vi "GRAPH.vi"() -> ()   [LabVIEW 2017]
uses:
  <vilib>/Utility/miscctls.llb/LVPointDoubleTypeDef.ctl
  <vilib>/measure/NI_MAPro.lvlib
panel:
  in  "peaks/valleys":u16(ring) items=["Peaks", "Valleys"]
  in  "width":i32=3
  out "# found":i32
  out "Array 2":ext[](array[numeric])
  in  "threshold":dbl=130.0 format="%#_13g"
  out "size(s) 3":i32
  out "2nd Derivatives":dbl[](array[numeric]) format="%0.2f"
  out "Amplitudes":dbl[](array[numeric]) format="%0.2f"
  out "Locations":dbl[](array[numeric]) format="%0.2f"
  out "time stamp":timestamp[](array[timestamp])
  out "XY Graph 2":cluster{"time stamp":timestamp, "X":dbl}[](graph)
  out "number":ext[](array[numeric])
  # "GRAPH"
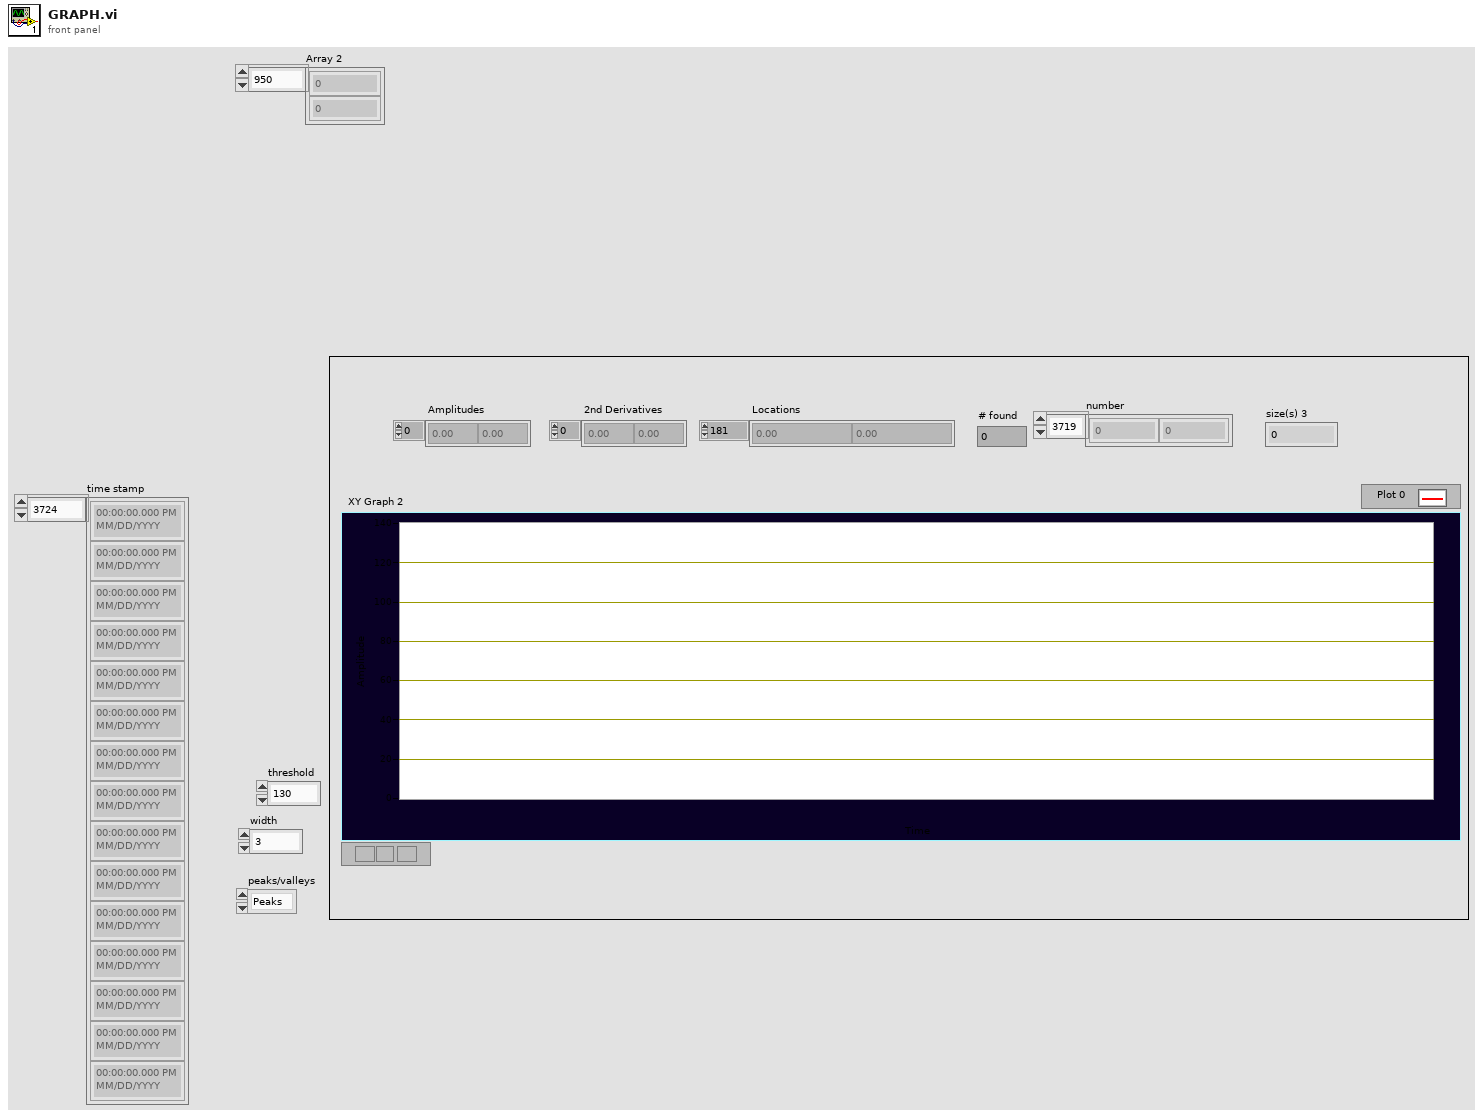
[diagram p1: front panel]
types:
  T1 = typedef "LVPointDoubleTypeDef.ctl" = cluster{"X":dbl, "Y":dbl}
  T2 = typedef "LVDateTimeRec.ctl" = cluster{"fractional second":dbl, "second":i32, "minute":i32, "hour":i32, "day of month":i32, "month":i32, "year":i32, "day of week":i32, "day of year":i32, "DST":i32}
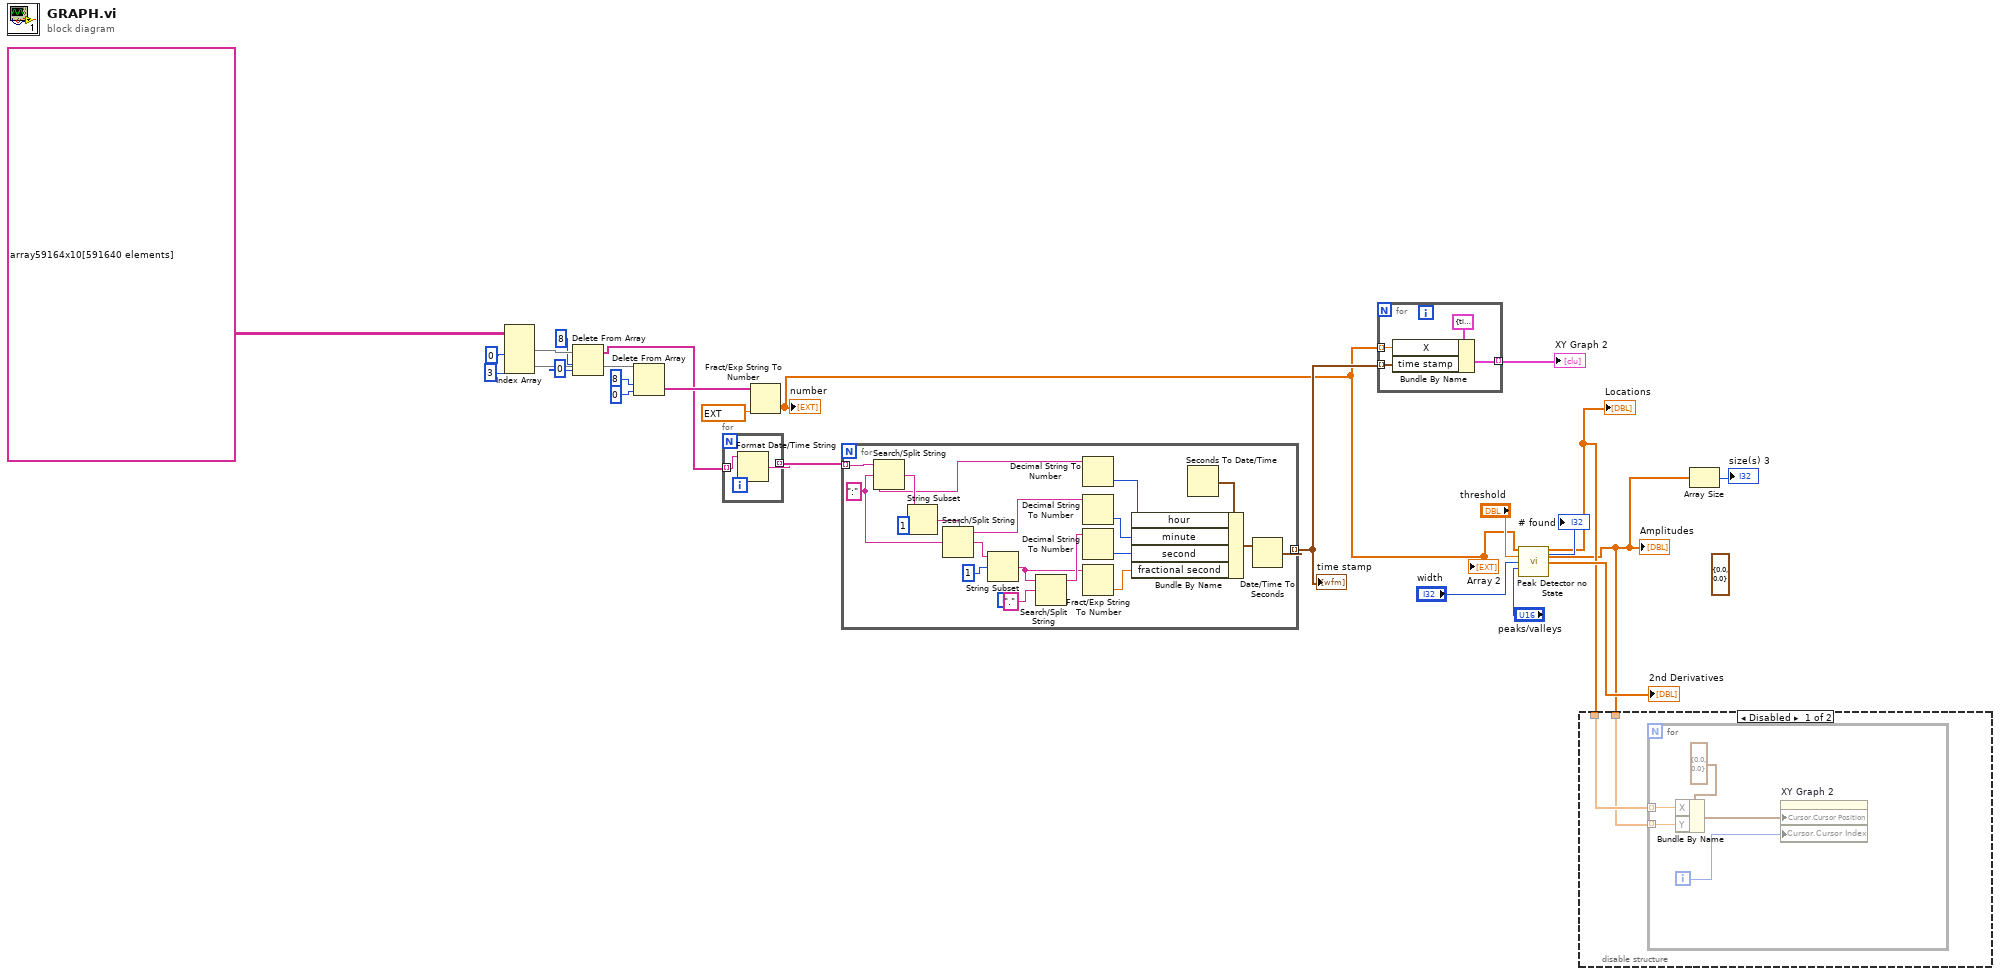
[diagram p0: block diagram]
diagram:
  (unwired) T1 {"X"=0.0, "Y"=0.0} ("Cursor.Cursor Position")
  n1 = Index Array(array=string[][] array59164x10[591640 elements] ("all rows 2"), index (col) #1=0 ("index (row)"), index (col) #2=3 ("disabled index (col)")) -> (element #1=w24:string[], element #2=w20:string[])  [unwired: 2 in]
  n2 = Delete From Array(array=w24, length=8 ("index (row)"), index=0 ("index (row)")) -> (array with subset deleted=w14:string[])  [unwired: 1 out]
  n3 = Delete From Array(array=w20, length=8 ("index (row)"), index=0 ("index (row)")) -> (array with subset deleted=w15:string[])  [unwired: 1 out]
  n4 = for {
    tunnel: w14 -> [w26] mode=indexing
    tunnel: [w25] -> w13 mode=indexing
    n5 = Format Date/Time String(time format string (%c)=w26) -> (date/time string=w25:string)  [unwired: 2 in]
  }
  n6 = Fract/Exp String To Number(string=w15, default (0 dbl)=ext 0.0 ("String")) -> (number=w5:ext[])  [unwired: 2 in, 1 out]
  "number" <- w5
  "Array 2" <- w5
  n7 = for {
    tunnel: w13 -> [w35] mode=indexing
    tunnel: [w43] -> w12 mode=indexing
    w42 = ":" ("format string")
    n8 = Search/Split String(string=w35, search string/char (-)=w42) -> (substring before match=w31:string, match + rest of string=w40:string)  [unwired: 1 in, 1 out]
    n9 = String Subset(string=w40, offset (0)=1) -> (substring=w39:string)  [unwired: 1 in]
    n10 = Search/Split String(string=w39, search string/char (-)=w42) -> (substring before match=w30:string, match + rest of string=w37:string)  [unwired: 1 in, 1 out]
    n11 = String Subset(string=w37, offset (0)=1) -> (substring=w29:string)  [unwired: 1 in]
    n12 = Search/Split String(string=w29, search string/char (-)="." ("format string")) -> (substring before match=w34:string)  [unwired: 1 in, 2 out]
    n13 = Decimal String To Number(string=w31) -> (number=w32:i32)  [unwired: 2 in, 1 out]
    n14 = Decimal String To Number(string=w30) -> (number=w33:i32)  [unwired: 2 in, 1 out]
    n15 = Decimal String To Number(string=w34) -> (number=w27:i32)  [unwired: 2 in, 1 out]
    n16 = Fract/Exp String To Number(string=w29) -> (number=w28:dbl)  [unwired: 3 in, 1 out]
    n17 = Seconds To Date/Time() -> (date time rec=w44:T2)  [unwired: 2 in]
    n18 = Bundle By Name(cluster=w44, "hour"=w32, "minute"=w33, "second"=w27, "fractional second"=w28) -> (w45:T2)
    n19 = Date/Time To Seconds(2:w45) -> (0:w43:timestamp)  [unwired: 1 in]
  }
  "time stamp" <- w12
  n20 = for {
    tunnel: w5 -> [w46] mode=indexing
    tunnel: [w49] -> w11 mode=indexing
    tunnel: w12 -> [w47] mode=indexing
    n21 = Bundle By Name(cluster=cluster{"time stamp":timestamp, "X":dbl} {"time stamp"=timestamp(0 s since 1904-01-01), "X"=0.0}, "X"=w46, "time stamp"=w47) -> (w49:cluster{"time stamp":timestamp, "X":dbl})
  }
  "XY Graph 2" <- w11
  n22 = call <vilib>:"Peak Detector no State.vi"("X"=w5, "threshold"="threshold", "width"="width", "peaks/valleys"="peaks/valleys") -> ("# found"=→"# found":i32, "Locations"=w3:dbl[], "Amplitudes"=w2:dbl[], "2nd Derivatives"=→"2nd Derivatives":dbl[])  [unwired: 4 in, 4 out]
  "Locations" <- w3
  "Amplitudes" <- w2
  n23 = disable-structure shown="Disabled" {
    disable-tunnel: w3 -> [w51 _]
    disable-tunnel: w2 -> [w50 _]
    frame Disabled {
      n24 = for {
        tunnel: w51 -> [w54] mode=indexing
        tunnel: w50 -> [w53] mode=indexing
        i -> [w52]
        n25 = Bundle By Name(cluster=T1 {"X"=0.0, "Y"=0.0} ("Cursor.Cursor Position"), "X"=w54, "Y"=w53) -> (w56:T1)
        n26 = property on="XY Graph 2" class="XYGraph (strict)"("Cursor.Cursor Position"=w56, "Cursor.Cursor Index"=w52) -> ()  [unwired: 2 in, 2 out]
      }
    }
    frame Enabled {
    }
  }
  n27 = Array Size(array=w2) -> (size(s)=→"size(s) 3":i32)
